vi "SR400 GetDiscParams.vi"(7 "error in (no error)":errorcluster, 10 "VISA Port In":refnum<visa-resource-name>="GPIB0::23::INSTR") -> (0 "error out":errorcluster, 1 "Discriminateur T":T1 {"Incrément (V)" min=-0.02 max=0.02 step=0.0002; "Niveau (V)" min=-0.3 max=0.3 step=0.0002; "Front A" items=["Montant", "Descendant"]; "Mode" items=["Fixe", "Scan"]}, 2 "Discriminateur B":T1 {"Incrément (V)" min=-0.02 max=0.02 step=0.0002; "Niveau (V)" min=-0.3 max=0.3 step=0.0002; "Front A" items=["Montant", "Descendant"]; "Mode" items=["Fixe", "Scan"]}, 3 "VISA Port Out":refnum<visa-resource-name>="SR400", 4 "Discriminateur A":T1 {"Incrément (V)" min=-0.02 max=0.02 step=0.0002; "Niveau (V)" min=-0.3 max=0.3 step=0.0002; "Front A" items=["Montant", "Descendant"]; "Mode" items=["Fixe", "Scan"]})   [LabVIEW 2019]
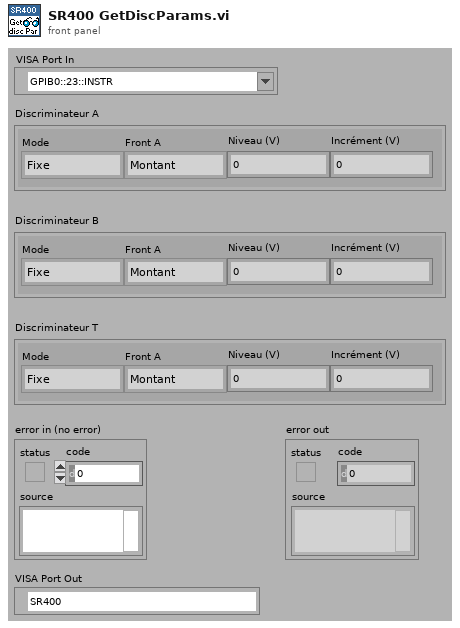
[diagram p1: front panel]
types:
  T1 = cluster{"Mode":u16, "Front A":u16, "Niveau (V)":dbl, "Incrément (V)":dbl}
  T2 = enum16{"Lit le Statut", "Demande Param", "Lit Param", "Oper. incomp."}
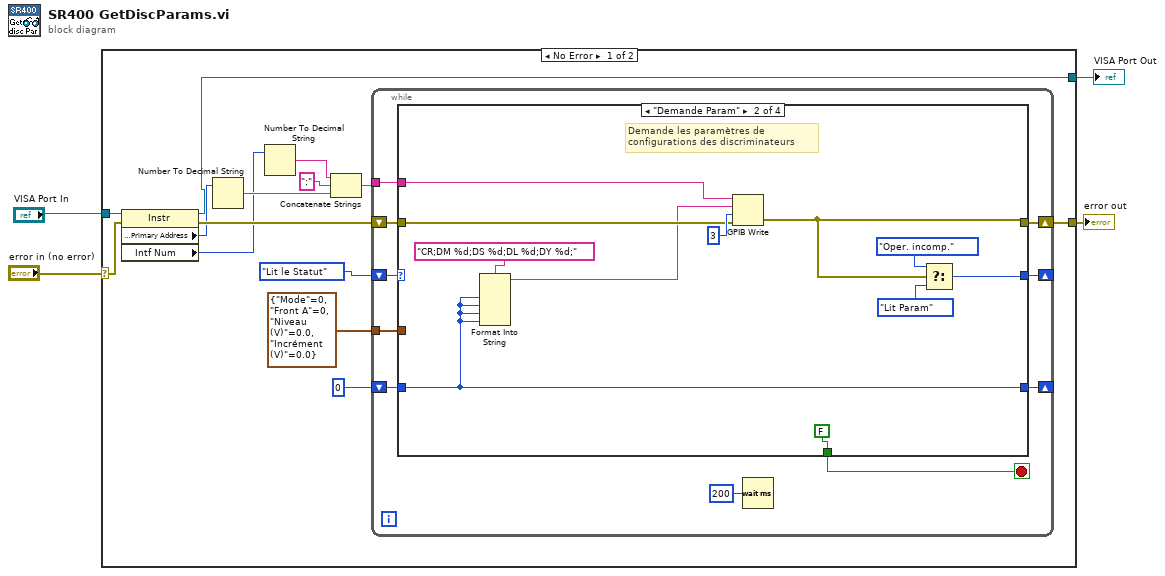
[diagram p0: block diagram]
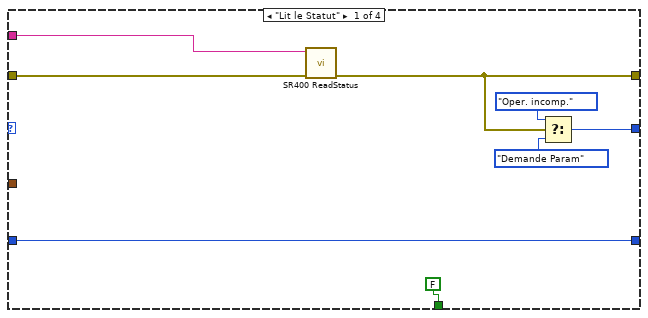
[diagram p2: hidden frame]
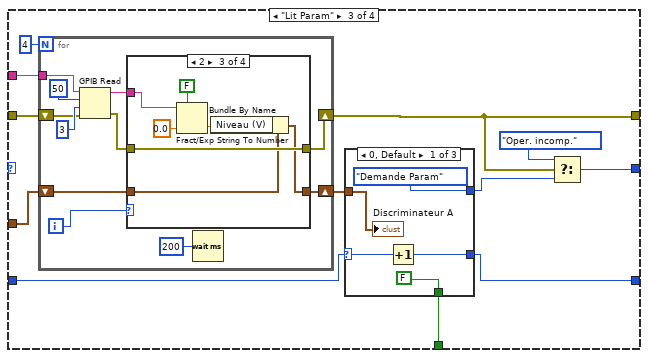
[diagram p3: hidden frame]
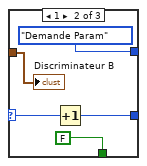
[diagram p4: hidden frame]
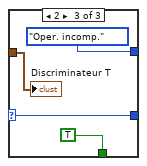
[diagram p5: hidden frame]
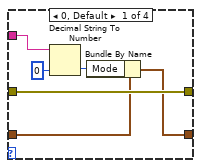
[diagram p6: hidden frame]
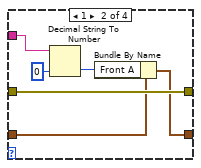
[diagram p7: hidden frame]
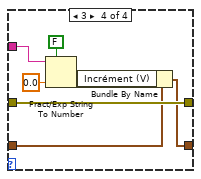
[diagram p8: hidden frame]
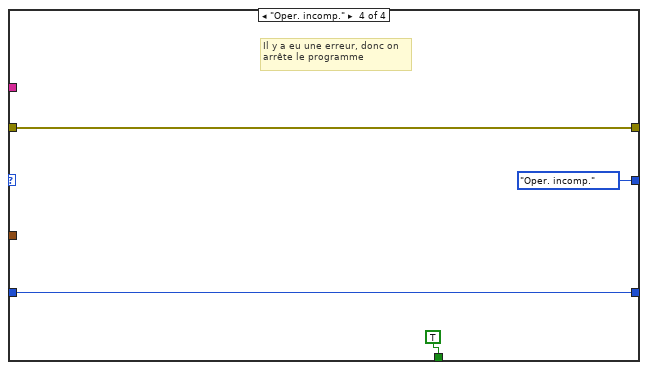
[diagram p9: hidden frame]
diagram:
  n1 = case shown="No Error" "error in (no error)" {
    selector: "error in (no error)" -> [w18 w116]
    tunnel: [w14 w116] -> w3
    tunnel: "VISA Port In" -> [w17 w115]
    tunnel: [w5 w115] -> w1
    frame No Error {
      n2 = property class="Instr"(reference=w17, error in=w18) -> (reference out=w5:refnum<visa-resource-name>, error out=w16:errorcluster, "GPIB Settings:Primary Address"=w15:u16, "Intf Num"=w6:u16)
      n3 = Number To Decimal String(number=w15) -> (decimal integer string=w9:string)  [unwired: 1 in]
      n4 = Number To Decimal String(number=w6) -> (decimal integer string=w8:string)  [unwired: 1 in]
      n5 = Concatenate Strings(w8, ":" ("string"), w9) -> (w10:string)
      n6 = while {
        shift-right: [w23] -> _
        shift-left: T2."Lit le Statut" -> [w28]
        tunnel: w10 -> [w26]
        shift-right: [w25] -> w14
        shift-left: w16 -> [w27]
        shift-right: [w20] -> _
        shift-left: 0 -> [w21]
        tunnel: T1 {"Mode"=0, "Front A"=0, "Niveau (V)"=0.0, "Incrément (V)"=0.0} ("Discriminateur B") -> [w19]
        stop <- w24 stop-if-true
        n7 = case shown="\"Demande Param\"" w28 {
          tunnel: w27 -> [w35 w45 w59 w114]
          tunnel: w26 -> [w34 w44 w58 _]
          tunnel: [w29 w37 w48 w114] -> w25
          tunnel: [FALSE ("Configuration\neffectuée") FALSE ("Configuration\neffectuée") w49 TRUE ("Configuration\neffectuée")] -> w24
          tunnel: [w33 w41 w51 T2."Oper. incomp."] -> w23
          tunnel: w21 -> [w30 w40 w55 w111]
          tunnel: [w30 w40 w53 w111] -> w20
          tunnel: w19 -> [_ _ w56 _]
          frame "Lit le Statut" {
            n8 = call <userlib>:"SR400 ReadStatus.vi"("error in"=w35, "Address string"=w34) -> ("Error Out"=w29:errorcluster)  [unwired: 6 in, 1 out]
            n9 = Select(t=T2."Oper. incomp.", s=w29, f=T2."Demande Param") -> (s? t:f=w33:T2)
          }
          frame "Demande Param" {
            # "Demande les paramètres de configurations des discriminateurs"
            n10 = Format Into String(format string="CR;DM %d;DS %d;DL %d;DY %d;", w40, w40, w40, w40) -> (resulting string=w38:string)  [unwired: 2 in, 1 out]
            n11 = GPIB Write(0:w44, 1:w38, 2:i16 3 ("mode (0)"), 3:w45) -> (6:w37:errorcluster)  [unwired: 1 in, 1 out]
            n12 = Select(t=T2."Oper. incomp.", s=w37, f=T2."Lit Param") -> (s? t:f=w41:T2)
          }
          frame "Lit Param" {
            n13 = for {
              N: 4 -> [_]
              shift-right: [w77] -> w48
              shift-left: w59 -> [w81]
              tunnel: w58 -> [w82]
              shift-right: [w76] -> w54
              shift-left: w56 -> [w75]
              i -> [w80]
              n14 = GPIB Read(0:w82, 1:50 ("byte count"), 2:i16 3 ("mode (0)"), 3:w81) -> (5:w78:string, 7:w79:errorcluster)  [unwired: 1 in, 1 out]
              n15 = case shown="2" w80 {
                tunnel: w79 -> [w88 w96 w103 w110]
                tunnel: w78 -> [w89 w94 w101 w105]
                tunnel: [w88 w96 w103 w110] -> w77
                tunnel: [w86 w92 w98 w106] -> w76
                tunnel: w75 -> [w85 w93 w99 w107]
                frame 0, Default {
                  n16 = Decimal String To Number(string=w89, default (0L)=u16 0 ("default (0 I32)")) -> (number=w87:u16)  [unwired: 1 in, 1 out]
                  n17 = Bundle By Name(cluster=w85, "Mode"=w87) -> (w86:T1)
                }
                frame 1 {
                  n18 = Decimal String To Number(string=w94, default (0L)=u16 0 ("default (0 I32)")) -> (number=w91:u16)  [unwired: 1 in, 1 out]
                  n19 = Bundle By Name(cluster=w93, "Front A"=w91) -> (w92:T1)
                }
                frame 2 {
                  n20 = Fract/Exp String To Number(use system decimal point (T)=FALSE, string=w101, default (0 dbl)=0.0 ("default (0 I32)")) -> (number=w100:dbl)  [unwired: 1 in, 1 out]
                  n21 = Bundle By Name(cluster=w99, "Niveau (V)"=w100) -> (w98:T1)
                }
                frame 3 {
                  n22 = Fract/Exp String To Number(use system decimal point (T)=FALSE, string=w105, default (0 dbl)=0.0 ("default (0 I32)")) -> (number=w108:dbl)  [unwired: 1 in, 1 out]
                  n23 = Bundle By Name(cluster=w107, "Incrément (V)"=w108) -> (w106:T1)
                }
              }
              n24 = Wait (ms)(milliseconds to wait=u32 200) -> ()  [unwired: 1 out]
            }
            n25 = case shown="0, Default" w55 {
              selector: w55 -> [w63 w68 w72]
              tunnel: w54 -> [w64 w69 w73]
              tunnel: [w62 w67 w72] -> w53
              tunnel: [T2."Demande Param" T2."Demande Param" T2."Oper. incomp."] -> w50
              tunnel: [FALSE ("Configuration\neffectuée") FALSE ("Configuration\neffectuée") TRUE ("Configuration\neffectuée")] -> w49
              frame 0, Default {
                n26 = Increment(x=w63) -> (x+1=w62:i32)
                "Discriminateur A" <- w64
              }
              frame 1 {
                n27 = Increment(x=w68) -> (x+1=w67:i32)
                "Discriminateur B" <- w69
              }
              frame 2 {
                "Discriminateur T" <- w73
              }
            }
            n28 = Select(t=T2."Oper. incomp.", s=w48, f=w50) -> (s? t:f=w51:T2)
          }
          frame "Oper. incomp." {
            # "Il y a eu une erreur, donc on arrête le programme"
          }
        }
        n29 = Wait (ms)(milliseconds to wait=u32 200) -> ()  [unwired: 1 out]
      }
    }
    frame Error {
    }
  }
  "error out" <- w3
  "VISA Port Out" <- w1
